vi "Parametric Curve Fitting - weighted.vi"() -> ()   [LabVIEW 2012]
doc: "This VI uses the Curve Fitting VIs to fit equations to curves and calculate confidence intervals.\n\nYou must select <B>Least Square</B> as the fitting <B>Method</B> to calculate the confidence interval of a fitted curve. The <B>Least Absolute Residual</B> and <B>Bisquare</B> fitting methods are less sensitive to outliers than the <B>Least Square</B> fitting method.\n\nNote: You can use this example only in the LabVIEW Full or Professional Development Systems."
uses:
  <vilib>/Analysis/6fits.llb/Confidence Interval (Linear).vi
  <vilib>/Analysis/6fits.llb/Confidence Interval (Exp).vi
  <vilib>/Analysis/6fits.llb/Confidence Interval (Power).vi
  <vilib>/Analysis/6fits.llb/Prediction Interval (Gauss).vi
  <vilib>/Analysis/6fits.llb/Confidence Interval (Log).vi
  <vilib>/Analysis/NI_AALPro.lvlib
panel:
  out "Observed Data and Fitted Curve  2":cluster{cluster{i32, dbl}[]}[](graph) caption="Observed Data and Fitted Curve"
  in  "polynomial order":i32=2
  in  "Weight":dbl[](array[numeric])
  in  "Intensity Data":dbl[](array[numeric])=[5.666666666666668, 2.666666666666668, -0.33333333333333215, 0.6666666666666679, -2.333333333333332, -5.333333333333332, -2.333333333333332, -4.333333333333332, -4.333333333333332, -0.33333333333333215, 0.6666666666666679, 2.666666666666668, 3.666666666666668, 12.666666666666668, 11.666666666666668, 16.666666666666668, 19.666666666666668, 25.666666666666668, 35.66666666666667, 46.66666666666667, 76.66666666666667, 119.66666666666667, 169.66666666666666, 227.66666666666666, 227.66666666666666, 227.66666666666666, 227.66666666666666, 227.66666666666666, 227.66666666666666, 130.66666666666666, 67.66666666666667, 26.666666666666668, 17.666666666666668, 11.666666666666668, 5.666666666666668, 4.666666666666668, 7.666666666666668, 4.666666666666668, 2.666666666666668, -2.333333333333332, -2.333333333333332, -3.333333333333332, -4.333333333333332, -3.333333333333332, -4.333333333333332, -2.333333333333332, -2.333333333333332, 0.6666666666666679, 0.6666666666666679, -0.33333333333333215]
  in  "confidence level":dbl=0.95 step=0.05 format="%_2g"
  out "Residue":dbl
  in  "Add outliers?":bool
  out "slope":dbl caption="Amplitude" format="%#.6g"
  out "Intercept":dbl caption="Center" format="%#.6g"
  in  "Tolerance":dbl=0.0001
  in  "Method":u16(ring) items=["Least Square", "Least Absolute Residual", "Bisquare"]
  in  "Data selector":T1(ring)=enum."Gaussian"
  out "Standard Deviation":dbl
  out "Observed Data and Fitted Curve":cluster{cluster{i32, "Numeric":dbl}[]}[](graph)
  # "Select Help>>Show Context Help and move the cursor over the VI icon to display help for this VI.\n\nInstructions:\n1) Run VI\n2) Select different parameters for the Data Input \nand Specifications\n3) Look at the block diagram for more information"
  # "Specifications"
  # "Results"
  # "Data Input"
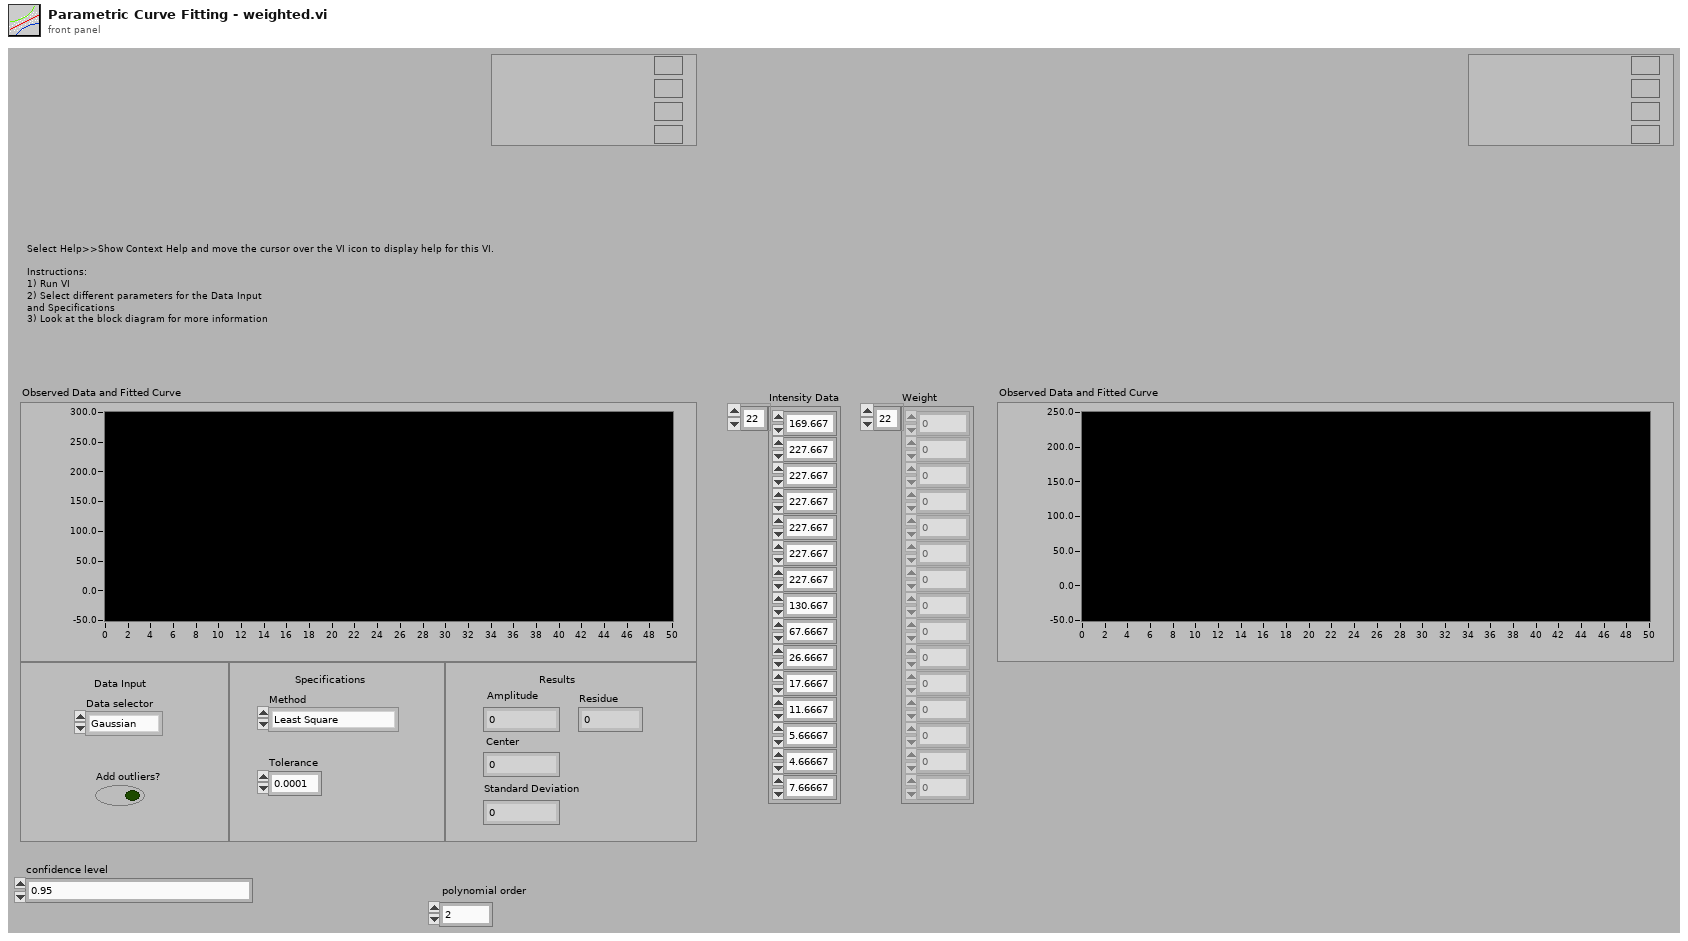
[diagram p1: front panel]
types:
  T1 = enum16{"Linear", "Exponential", "Power", "Gaussian", "Logarithmic"}
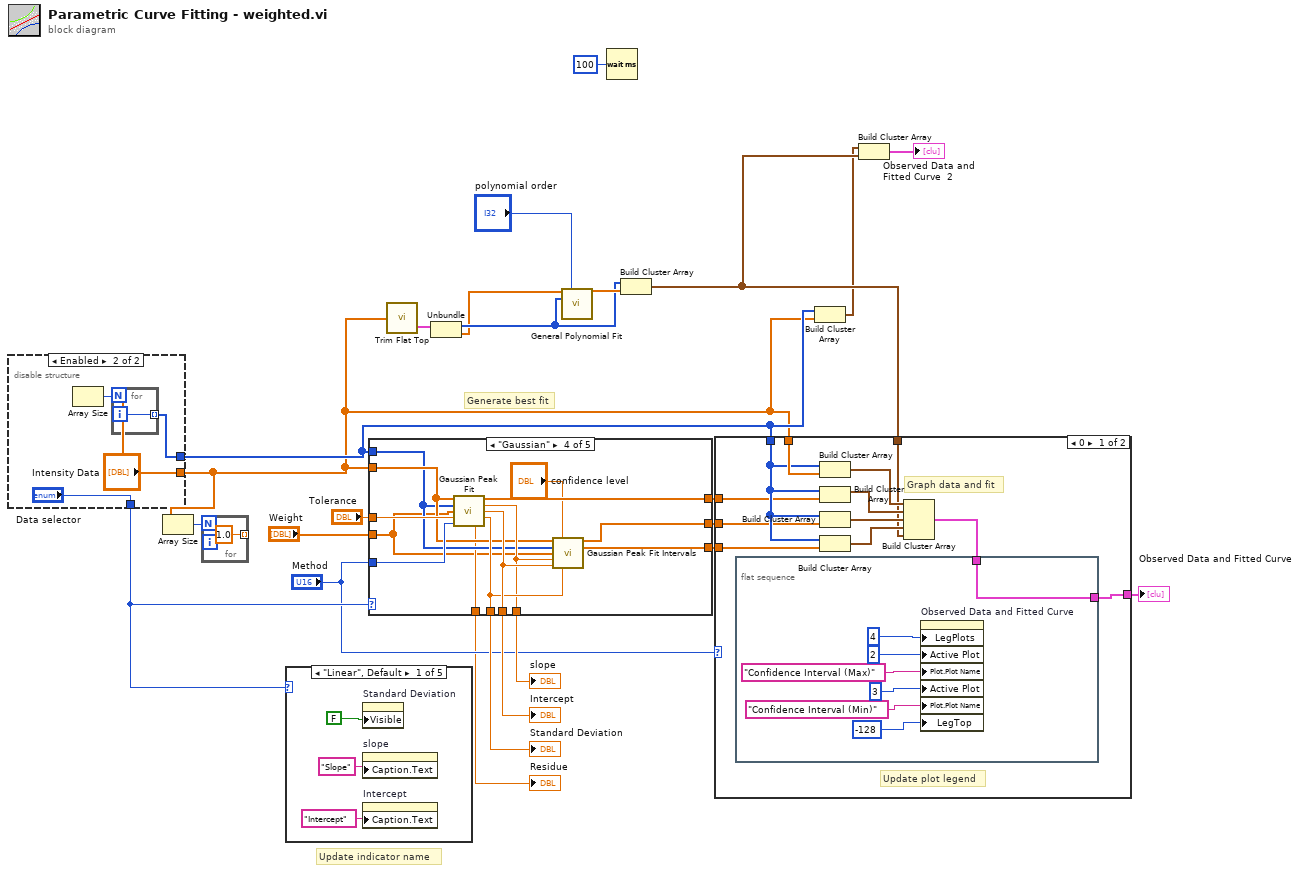
[diagram p0: block diagram]
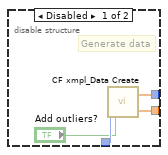
[diagram p2: hidden frame]
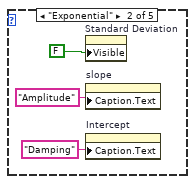
[diagram p3: hidden frame]
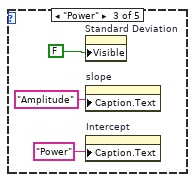
[diagram p4: hidden frame]
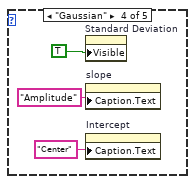
[diagram p5: hidden frame]
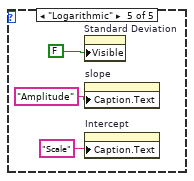
[diagram p6: hidden frame]
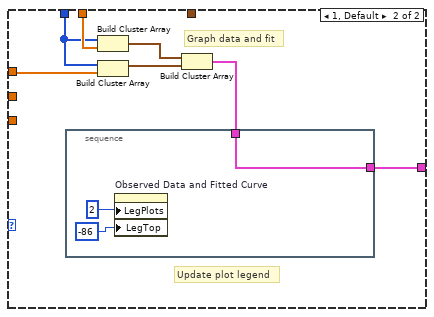
[diagram p7: hidden frame]
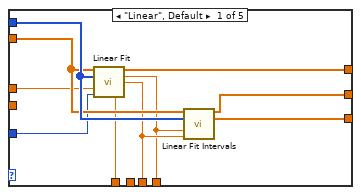
[diagram p8: hidden frame]
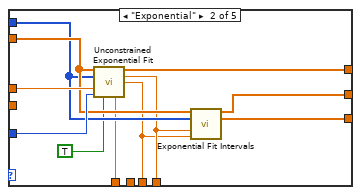
[diagram p9: hidden frame]
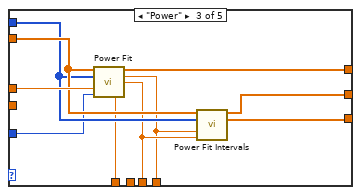
[diagram p10: hidden frame]
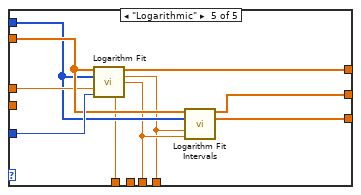
[diagram p11: hidden frame]
diagram:
  # "Update indicator name"
  # "Generate best fit"
  n1 = disable-structure shown="Enabled" {
    disable-tunnel: [w28 w30] -> w4
    disable-tunnel: [w27 "Intensity Data"] -> w3
    disable-tunnel: [w26 "Data selector"] -> w17
    frame Disabled {
      # "Generate data"
      n2 = call "CF xmpl_Data Create.vi"("Add outliers?"="Add outliers?") -> ("Y"=w27:dbl[], "X"=w28:dbl[], "Signal type"=w26:T1)
    }
    frame Enabled {
      n3 = Array Size(array="Intensity Data") -> (size(s)=w32:i32)
      n4 = for {
        N: w32 -> [_]
        tunnel: [w33] -> w30 mode=indexing
        i -> [w33]
      }
    }
  }
  n5 = Array Size(array=w3) -> (size(s)=w13:i32)
  n6 = for {
    N: w13 -> [_]
    tunnel: [1.0] -> _ mode=indexing
  }
  n7 = case shown="\"Linear\", Default" w17 {
    frame "Linear", Default {
      n8 = property on="Standard Deviation" class="DigNum (strict)"("Visible"=FALSE) -> ()  [unwired: 2 in, 2 out]
      n9 = property on="slope" class="DigNum (strict)"("Caption.Text"="Slope" ("Label.Text")) -> ()  [unwired: 2 in, 2 out]
      n10 = property on="Intercept" class="DigNum (strict)"("Caption.Text"="Intercept") -> ()  [unwired: 2 in, 2 out]
    }
    frame "Exponential" {
      n11 = property on="Standard Deviation" class="DigNum (strict)"("Visible"=FALSE) -> ()  [unwired: 2 in, 2 out]
      n12 = property on="slope" class="DigNum (strict)"("Caption.Text"="Amplitude" ("Label.Text")) -> ()  [unwired: 2 in, 2 out]
      n13 = property on="Intercept" class="DigNum (strict)"("Caption.Text"="Damping") -> ()  [unwired: 2 in, 2 out]
    }
    frame "Power" {
      n14 = property on="Standard Deviation" class="DigNum (strict)"("Visible"=FALSE) -> ()  [unwired: 2 in, 2 out]
      n15 = property on="slope" class="DigNum (strict)"("Caption.Text"="Amplitude" ("Label.Text")) -> ()  [unwired: 2 in, 2 out]
      n16 = property on="Intercept" class="DigNum (strict)"("Caption.Text"="Power") -> ()  [unwired: 2 in, 2 out]
    }
    frame "Gaussian" {
      n17 = property on="Standard Deviation" class="DigNum (strict)"("Visible"=TRUE) -> ()  [unwired: 2 in, 2 out]
      n18 = property on="slope" class="DigNum (strict)"("Caption.Text"="Amplitude" ("Label.Text")) -> ()  [unwired: 2 in, 2 out]
      n19 = property on="Intercept" class="DigNum (strict)"("Caption.Text"="Center") -> ()  [unwired: 2 in, 2 out]
    }
    frame "Logarithmic" {
      n20 = property on="Standard Deviation" class="DigNum (strict)"("Visible"=FALSE) -> ()  [unwired: 2 in, 2 out]
      n21 = property on="slope" class="DigNum (strict)"("Caption.Text"="Amplitude" ("Label.Text")) -> ()  [unwired: 2 in, 2 out]
      n22 = property on="Intercept" class="DigNum (strict)"("Caption.Text"="Scale") -> ()  [unwired: 2 in, 2 out]
    }
  }
  n23 = case shown="\"Gaussian\"" w17 {
    tunnel: [w59 w64 w77 w91 w101] -> w21
    tunnel: [w58 w65 w75 w92 w103] -> w23
    tunnel: [w57 w66 w76 w81 w102] -> w22
    tunnel: w4 -> [w56 w67 w78 w85 w97]
    tunnel: w3 -> [w55 w68 w79 w86 w99]
    tunnel: "Tolerance" -> [w54 w70 w80 w93 w98]
    tunnel: "Method" -> [w53 w69 w74 w90 w100]
    tunnel: [w52 w61 w73 w89 w96] -> w19
    tunnel: [w51 w62 w72 w87 w95] -> w20
    tunnel: [_ _ _ w88 _] -> w18
    tunnel: [w50 w60 w71 w84 w94] -> w14
    tunnel: "Weight" -> [_ _ _ w82 _]
    frame "Linear", Default {
      n24 = call <vilib>:"Linear Fit.vi"("Y"=w55, "X"=w56, "tolerance"=w54, "method"=w53) -> ("Best Linear Fit"=w59:dbl[], "slope"=w51:dbl, "intercept"=w52:dbl, "residue"=w50:dbl)  [unwired: 7 in, 1 out]
      n25 = call-poly <vilib>:"Linear Fit Intervals.vi"("Y"=w55, "X"=w56, "slope"=w51, "intercept"=w52) -> ("Upper Bound"=w57:dbl[], "Lower Bound"=w58:dbl[])  [unwired: 7 in, 3 out]
    }
    frame "Exponential" {
      n26 = call <vilib>:"Unconstrained Exponential Fit.vi"("Y"=w68, "X"=w67, "tolerance"=w70, "method"=w69, "refine?"=TRUE) -> ("Best Exponential Fit"=w64:dbl[], "amplitude"=w62:dbl, "damping"=w61:dbl, "residue"=w60:dbl)  [unwired: 6 in, 1 out]
      n27 = call-poly <vilib>:"Exponential Fit Intervals.vi"("Y"=w68, "X"=w67, "amplitude"=w62, "damping"=w61) -> ("Upper Bound"=w66:dbl[], "Lower Bound"=w65:dbl[])  [unwired: 7 in, 3 out]
    }
    frame "Power" {
      n28 = call <vilib>:"Power Fit.vi"("Y"=w79, "X"=w78, "tolerance"=w80, "method"=w74) -> ("Best Power Fit"=w77:dbl[], "amplitude"=w72:dbl, "power"=w73:dbl, "residue"=w71:dbl)  [unwired: 6 in, 2 out]
      n29 = call-poly <vilib>:"Power Fit Intervals.vi"("Y"=w79, "X"=w78, "amplitude"=w72, "power"=w73) -> ("Upper Bound"=w76:dbl[], "Lower Bound"=w75:dbl[])  [unwired: 7 in, 3 out]
    }
    frame "Gaussian" {
      n30 = call <vilib>:"Gaussian Peak Fit.vi"("Y"=w86, "X"=w85, "Weight"=w82, "tolerance"=w93, "method"=w90) -> ("Best Gaussian Fit"=w91:dbl[], "amplitude"=w87:dbl, "center"=w89:dbl, "standard deviation"=w88:dbl, "residue"=w84:dbl)  [unwired: 4 in, 2 out]
      n31 = call-poly <vilib>:"Gaussian Peak Fit Intervals.vi"("Y"=w86, "confidence level"="confidence level", "X"=w85, "Weight"=w82, "amplitude"=w87, "center"=w89, "standard deviation"=w88) -> ("Upper Bound"=w81:dbl[], "Lower Bound"=w92:dbl[])  [unwired: 6 in, 1 out]
    }
    frame "Logarithmic" {
      n32 = call <vilib>:"Logarithm Fit.vi"("Y"=w99, "X"=w97, "tolerance"=w98, "method"=w100) -> ("Best Logarithm Fit"=w101:dbl[], "amplitude"=w95:dbl, "scale"=w96:dbl, "residue"=w94:dbl)  [unwired: 7 in, 1 out]
      n33 = call-poly <vilib>:"Logarithm Fit Intervals.vi"("Y"=w99, "X"=w97, "amplitude"=w95, "scale"=w96) -> ("Upper Bound"=w102:dbl[], "Lower Bound"=w103:dbl[])  [unwired: 7 in, 3 out]
    }
  }
  "slope" <- w20
  "Intercept" <- w19
  "Standard Deviation" <- w18
  "Residue" <- w14
  n34 = call "Trim Flat Top.vi"("Data In"=w3) -> ("Trimmed Data (x,y)"=w8:cluster{i32[], dbl[]})  [unwired: 1 out]
  n35 = Unbundle(w8) -> (w7:i32[], w6:dbl[])
  n36 = call <vilib>:"General Polynomial Fit.vi"("Y"=w6, "polynomial order"="polynomial order", "X"=w7) -> ("Best Polynomial Fit"=w10:dbl[])  [unwired: 9 in, 3 out]
  n37 = Wait (ms)(milliseconds to wait=u32 100) -> ()  [unwired: 1 out]
  n38 = Build Cluster Array(w7, w10) -> (w5:cluster{i32, dbl}[])
  n39 = case shown="0" "Method" {
    tunnel: w3 -> [w111 w126]
    tunnel: w4 -> [w110 w125]
    tunnel: w23 -> [w109 _]
    tunnel: w22 -> [w108 _]
    tunnel: w21 -> [w107 w127]
    tunnel: [w105 w123] -> w15
    tunnel: w5 -> [w104 _]
    frame 0 {
      # "Graph data and fit"
      # "Update plot legend"
      n40 = flat-sequence {
        tunnel: w106 -> [w122]
        tunnel: [w122] -> w105
        frame #0 {
          n41 = property on="Observed Data and Fitted Curve" class="XYGraph (strict)"("LegPlots"=u32 4 ("Legend:Plots Shown"), "Active Plot"=u32 2, "Plot.Plot Name"="Confidence Interval (Max)", "Active Plot"=u32 3, "Plot.Plot Name"="Confidence Interval (Min)", "LegTop"=-128 ("Legend:Position:Top")) -> ()  [unwired: 2 in, 2 out]
        }
      }
      n42 = Build Cluster Array(w110, w111) -> (w113:cluster{i32, dbl}[])
      n43 = Build Cluster Array(w110, w107) -> (w112:cluster{i32, "Numeric":dbl}[])
      n44 = Build Cluster Array(w110, w108) -> (w115:cluster{i32, "Numeric":dbl}[])
      n45 = Build Cluster Array(w110, w109) -> (w114:cluster{i32, "Numeric":dbl}[])
      n46 = Build Cluster Array(w113, w112, w115, w114, w104) -> (w106:cluster{cluster{i32, "Numeric":dbl}[]}[])
    }
    frame 1, Default {
      # "Update plot legend"
      # "Graph data and fit"
      n47 = Build Cluster Array(w125, w126) -> (w129:cluster{i32, dbl}[])
      n48 = Build Cluster Array(w125, w127) -> (w128:cluster{i32, "Numeric":dbl}[])
      n49 = Build Cluster Array(w129, w128) -> (w124:cluster{cluster{i32, "Numeric":dbl}[]}[])
      n50 = stacked-sequence {
        tunnel: w124 -> [w131]
        tunnel: [w131] -> w123
        frame #0 {
          n51 = property on="Observed Data and Fitted Curve" class="XYGraph (strict)"("LegPlots"=u32 2 ("Legend:Plots Shown"), "LegTop"=-86 ("Legend:Position:Top")) -> ()  [unwired: 2 in, 2 out]
        }
      }
    }
  }
  "Observed Data and Fitted Curve" <- w15
  n52 = Build Cluster Array(w4, w3) -> (w2:cluster{i32, dbl}[])
  n53 = Build Cluster Array(w2, w5) -> (→"Observed Data and Fitted Curve  2":cluster{cluster{i32, dbl}[]}[])
